vi "Add Metadata.vi"(8 "error in (no error)":errorcluster, 9 "Reset":bool, 10 "Metadata":refnum<class "Metadata.lvclass">[](array[class]), 11 "Worker in":refnum<class "Worker.lvclass">) -> (0 "error out":errorcluster, 3 "Worker out":refnum<class "Worker.lvclass">)   [LabVIEW 2020, in "Worker.lvclass"]
uses:
  Worker.lvclass
  NHMFL_Core/Libraries/File/Metadata/Metadata.lvclass
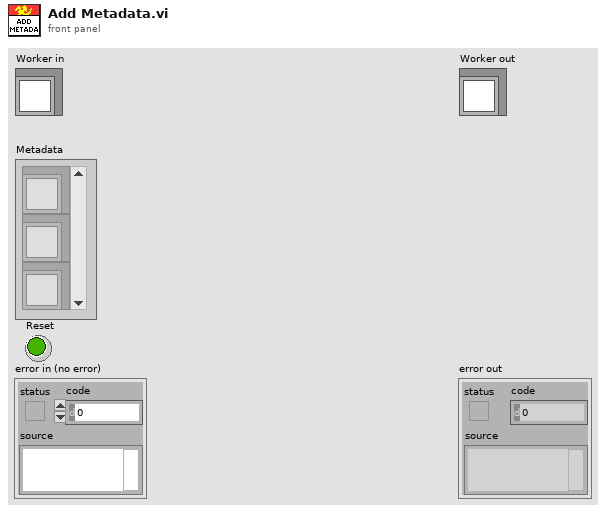
[diagram p1: front panel]
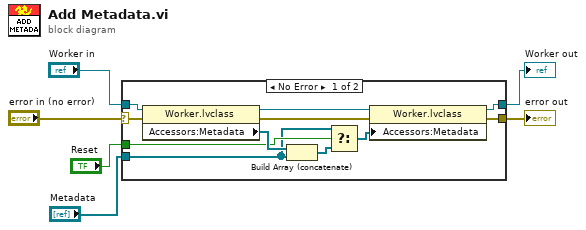
[diagram p0: block diagram]
diagram:
  n1 = case shown="No Error" "error in (no error)" {
    selector: "error in (no error)" -> [w17 w19]
    tunnel: [w14 w19] -> w5
    tunnel: [w12 w18] -> w3
    tunnel: "Worker in" -> [w15 w18]
    tunnel: "Metadata" -> [w9 _]
    tunnel: "Reset" -> [w10 _]
    frame No Error {
      n2 = property class="Worker.lvclass"(reference=w15, error in=w17) -> (reference out=w13:refnum<class "Worker.lvclass">, error out=w16:errorcluster, "Accessors:Metadata"=w11:refnum<class "Metadata.lvclass">[])
      n3 = Build Array (concatenate)(w11, w9) -> (w8:refnum<class "Metadata.lvclass">[])
      n4 = Select(t=w9, s=w10, f=w8) -> (s? t:f=w7:refnum<class "Metadata.lvclass">[])
      n5 = property class="Worker.lvclass"(reference=w13, error in=w16, "Accessors:Metadata"=w7) -> (reference out=w12:refnum<class "Worker.lvclass">, error out=w14:errorcluster)
    }
    frame Error {
    }
  }
  "error out" <- w5
  "Worker out" <- w3
